vi "update Rows.vi"(8 "error in (no error)":errorcluster, 10 "Cells":T2(array[cluster]), 11 "DataGridView in":refnum<class "DataGridView.lvclass">) -> (0 "error out":errorcluster, 3 "DataGridView out":refnum<class "DataGridView.lvclass">)   [LabVIEW 2013, in "DataGrid.lvlib" / "DataGridView.lvclass"]
doc: "This method allows you to add any rows of any time, regardless of the data column setup."
uses:
  DataGridView.lvclass
  GridColumn/ColumnType.ctl
  DataGridView.lvclass/DataGridView.ctl
  System.Windows.Forms
  DataTable/DataTable.lvclass
  GridColumn/GridColumn.lvclass
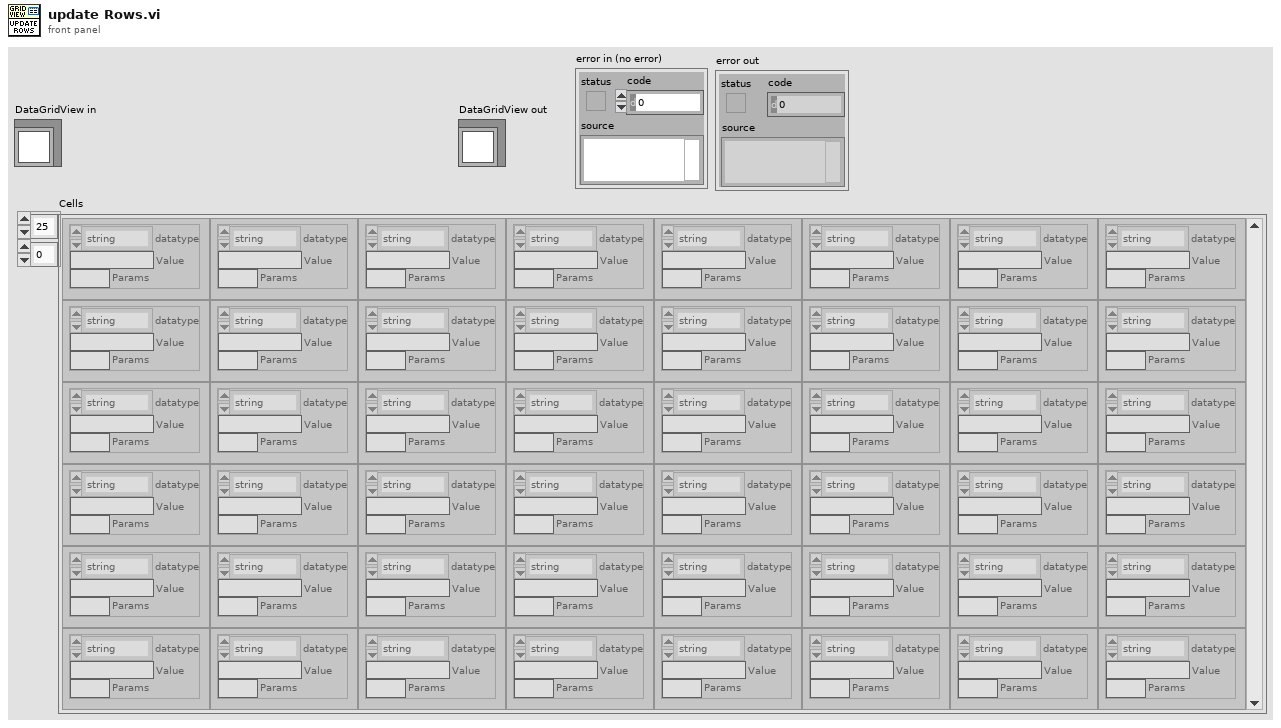
[diagram p1: front panel]
types:
  T1 = typedef "DataGrid.lvlib/GridColumn.lvclass/ColumnType.ctl" = enum16{"string", "image", "check", "numeric", "timestamp", "button", "combo", "link"}
  T2 = cluster{"datatype":T1, "Value":string, "Params":string}[][]
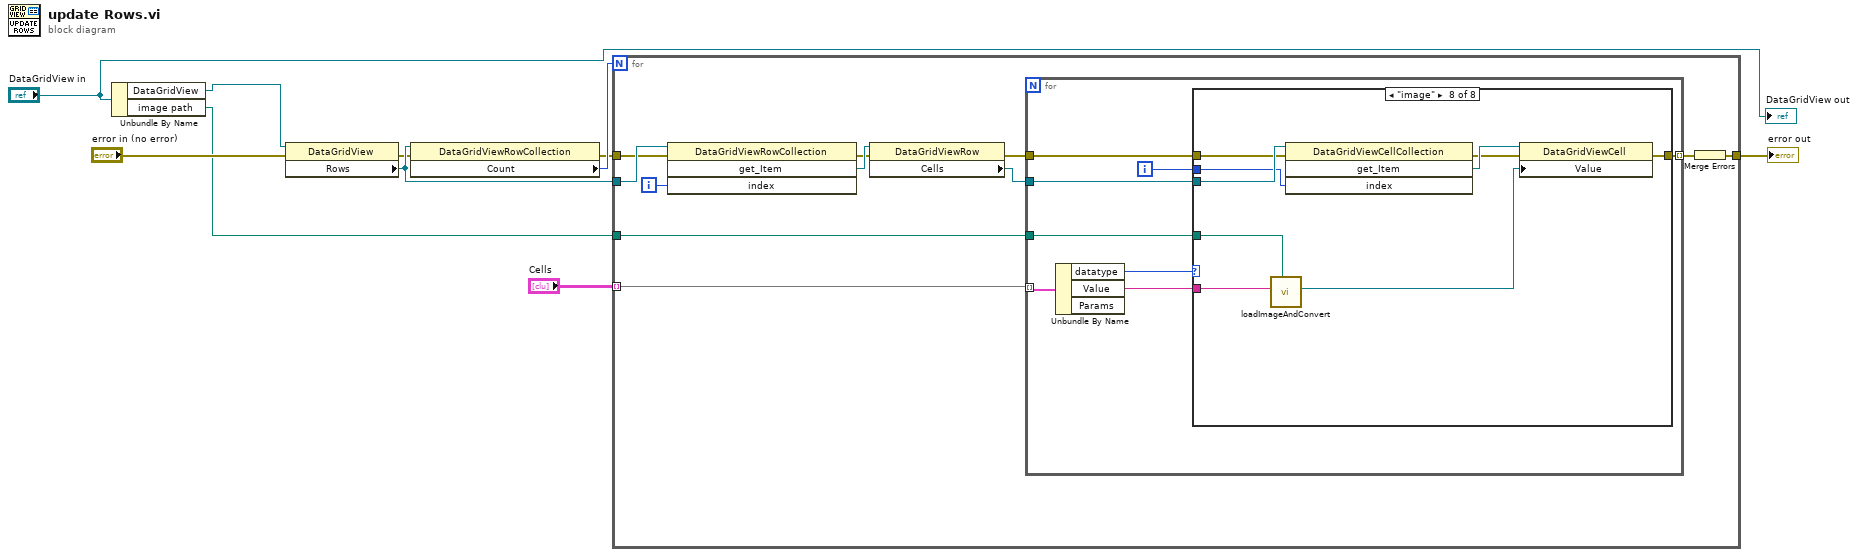
[diagram p0: block diagram]
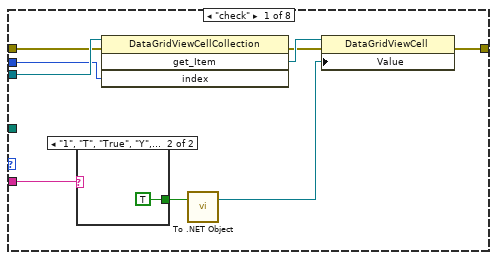
[diagram p2: hidden frame]
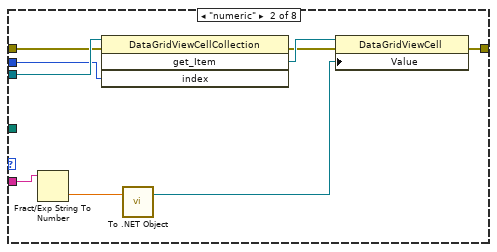
[diagram p4: hidden frame]
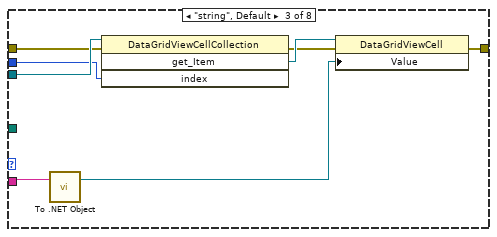
[diagram p5: hidden frame]
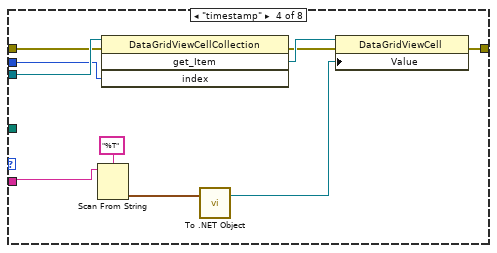
[diagram p6: hidden frame]
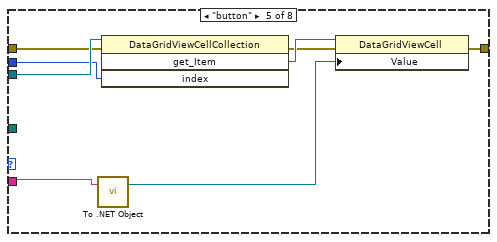
[diagram p7: hidden frame]
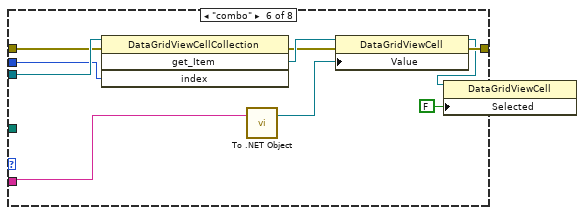
[diagram p8: hidden frame]
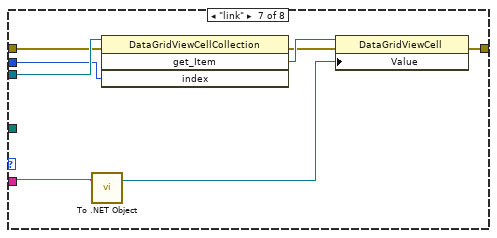
[diagram p9: hidden frame]
diagram:
  n1 = Unbundle By Name("DataGridView in") -> ("DataGridView"=w5:refnum<k24>, "image path"=w3:path)
  n2 = property class="DataGridView"(reference=w5, error in="error in (no error)") -> (error out=w8:errorcluster, "Rows"=w10:refnum<k24>)  [unwired: 1 out]
  n3 = property class="DataGridViewRowCollection"(reference=w10, error in=w8) -> (error out=w7:errorcluster, "Count"=w9:i32)  [unwired: 1 out]
  n4 = for {
    N: w9 -> [_]
    tunnel: w10 -> [w21]
    tunnel: w7 -> [w17]
    tunnel: [w14] -> w2
    tunnel: "Cells" -> [w11] mode=indexing
    tunnel: w3 -> [w12]
    i -> [w20]
    n5 = invoke class="DataGridViewRowCollection" method="get_Item"(reference=w21, error in=w17, "index"=w20) -> (error out=w16:errorcluster, "get_Item"=w19:refnum<k24>)  [unwired: 1 in, 2 out]
    n6 = property class="DataGridViewRow"(reference=w19, error in=w16) -> (error out=w13:errorcluster, "Cells"=w18:refnum<k24>)  [unwired: 1 out]
    n7 = for {
      tunnel: w18 -> [w29]
      tunnel: w13 -> [w27]
      tunnel: [w26] -> w15 mode=indexing
      tunnel: w11 -> [w25] mode=indexing
      tunnel: w12 -> [w22]
      i -> [w28]
      n8 = Unbundle By Name(w25) -> ("datatype"=w24:T1, "Value"=w23:string)  [unwired: 1 out]
      n9 = case shown="\"image\"" w24 {
        tunnel: w29 -> [w38 w48 w56 w66 w74 w84 w92 w101]
        tunnel: w28 -> [w37 w47 w55 w65 w73 w83 w91 w100]
        tunnel: w27 -> [w36 w46 w54 w64 w72 w82 w90 w99]
        tunnel: [w30 w40 w51 w61 w69 w79 w87 w96] -> w26
        tunnel: w23 -> [w32 w42 w50 w58 w68 w78 w86 w95]
        tunnel: w22 -> [_ _ _ _ _ _ _ w94]
        frame "check" {
          n10 = case shown="\"1\", \"T\", \"True\", \"Y\", \"Yes\"" w32 {
            tunnel: [_ TRUE] -> w33
            frame Default {
            }
            frame "1", "T", "True", "Y", "Yes" {
            }
          }
          n11 = invoke class="DataGridViewCellCollection" method="get_Item"(reference=w38, error in=w36, "index"=w37) -> (error out=w34:errorcluster, "get_Item"=w35:refnum<k24>)  [unwired: 1 in, 2 out]
          n12 = call <vilib>:"To .NET Object.vi"("anything"=w33) -> (".NET object"=w31:refnum<k24>)  [unwired: 1 in, 1 out]
          n13 = property class="DataGridViewCell"(reference=w35, error in=w34, "Value"=w31) -> (error out=w30:errorcluster)  [unwired: 1 out]
        }
        frame "numeric" {
          n14 = Fract/Exp String To Number(string=w42) -> (number=w43:dbl)  [unwired: 3 in, 1 out]
          n15 = invoke class="DataGridViewCellCollection" method="get_Item"(reference=w48, error in=w46, "index"=w47) -> (error out=w44:errorcluster, "get_Item"=w45:refnum<k24>)  [unwired: 1 in, 2 out]
          n16 = call <vilib>:"To .NET Object.vi"("anything"=w43) -> (".NET object"=w41:refnum<k24>)  [unwired: 1 in, 1 out]
          n17 = property class="DataGridViewCell"(reference=w45, error in=w44, "Value"=w41) -> (error out=w40:errorcluster)  [unwired: 1 out]
        }
        frame "string", Default {
          n18 = call <vilib>:"To .NET Object.vi"("anything"=w50) -> (".NET object"=w49:refnum<k24>)  [unwired: 1 in, 1 out]
          n19 = invoke class="DataGridViewCellCollection" method="get_Item"(reference=w56, error in=w54, "index"=w55) -> (error out=w52:errorcluster, "get_Item"=w53:refnum<k24>)  [unwired: 1 in, 2 out]
          n20 = property class="DataGridViewCell"(reference=w53, error in=w52, "Value"=w49) -> (error out=w51:errorcluster)  [unwired: 1 out]
        }
        frame "timestamp" {
          n21 = Scan From String(format string="%T", input string=w58) -> (output 1=w60:timestamp)  [unwired: 3 in, 3 out]
          n22 = invoke class="DataGridViewCellCollection" method="get_Item"(reference=w66, error in=w64, "index"=w65) -> (error out=w62:errorcluster, "get_Item"=w63:refnum<k24>)  [unwired: 1 in, 2 out]
          n23 = call <vilib>:"To .NET Object.vi"("anything"=w60) -> (".NET object"=w57:refnum<k24>)  [unwired: 1 in, 1 out]
          n24 = property class="DataGridViewCell"(reference=w63, error in=w62, "Value"=w57) -> (error out=w61:errorcluster)  [unwired: 1 out]
        }
        frame "button" {
          n25 = call <vilib>:"To .NET Object.vi"("anything"=w68) -> (".NET object"=w67:refnum<k24>)  [unwired: 1 in, 1 out]
          n26 = invoke class="DataGridViewCellCollection" method="get_Item"(reference=w74, error in=w72, "index"=w73) -> (error out=w70:errorcluster, "get_Item"=w71:refnum<k24>)  [unwired: 1 in, 2 out]
          n27 = property class="DataGridViewCell"(reference=w71, error in=w70, "Value"=w67) -> (error out=w69:errorcluster)  [unwired: 1 out]
        }
        frame "combo" {
          n28 = invoke class="DataGridViewCellCollection" method="get_Item"(reference=w84, error in=w82, "index"=w83) -> (error out=w80:errorcluster, "get_Item"=w81:refnum<k24>)  [unwired: 1 in, 2 out]
          n29 = call <vilib>:"To .NET Object.vi"("anything"=w78) -> (".NET object"=w77:refnum<k24>)  [unwired: 1 in, 1 out]
          n30 = property class="DataGridViewCell"(reference=w81, error in=w80, "Value"=w77) -> (reference out=w76:refnum<k24>, error out=w79:errorcluster)
          n31 = property class="DataGridViewCell"(reference=w76, "Selected"=FALSE) -> ()  [unwired: 1 in, 2 out]
        }
        frame "link" {
          n32 = call <vilib>:"To .NET Object.vi"("anything"=w86) -> (".NET object"=w85:refnum<k24>)  [unwired: 1 in, 1 out]
          n33 = invoke class="DataGridViewCellCollection" method="get_Item"(reference=w92, error in=w90, "index"=w91) -> (error out=w88:errorcluster, "get_Item"=w89:refnum<k24>)  [unwired: 1 in, 2 out]
          n34 = property class="DataGridViewCell"(reference=w89, error in=w88, "Value"=w85) -> (error out=w87:errorcluster)  [unwired: 1 out]
        }
        frame "image" {
          n35 = call "loadImageAndConvert.vi"("image path"=w94, "name or relative path"=w95) -> (".NET object"=w93:refnum<k24>)  [unwired: 8 in, 1 out]
          n36 = invoke class="DataGridViewCellCollection" method="get_Item"(reference=w101, error in=w99, "index"=w100) -> (error out=w97:errorcluster, "get_Item"=w98:refnum<k24>)  [unwired: 1 in, 2 out]
          n37 = property class="DataGridViewCell"(reference=w98, error in=w97, "Value"=w93) -> (error out=w96:errorcluster)  [unwired: 1 out]
        }
      }
    }
    n38 = Merge Errors(w15) -> (w14:errorcluster)
  }
  "error out" <- w2
  "DataGridView out" <- "DataGridView in"
